vi "Agilent VNA Read Trace Display.vi"(4 "Trace":i8=1 min=1 max=99 step=1, 6 "Channel":i8=1 min=1 max=99 step=1, 7 "Agilent VNA":T1, 8 "error in (no error)":errorcluster, 11 "VISA Resource Name":refnum<visa-resource-name>) -> (0 "error out":errorcluster, 1 "Measurements":string[](array[string]), 2 "Displayed?":bool, 3 "dup VISA Resource Name":refnum<visa-resource-name>)   [LabVIEW 2011]
uses:
  TypeDefs/Agilent VNA Instrument Info.ctl
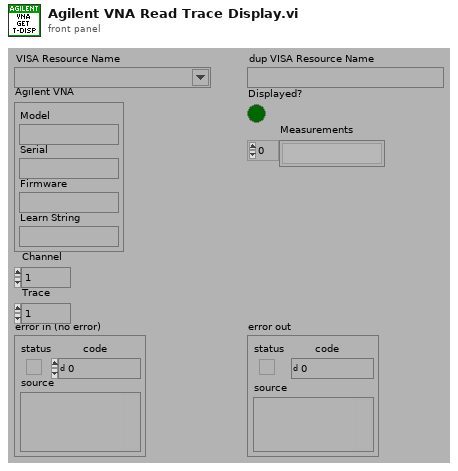
[diagram p1: front panel]
types:
  T1 = typedef "Agilent VNA Instrument Info.ctl" = cluster{"Model":string, "Serial":string, "Firmware":string, "Learn String":string}
  T2 = typedef "Agilent VNA Model.ctl" = enum16{"Not Supported", "8510X", "8719X", "8720X", "8722X", "8753X", "ENA", "PNA", "Field Fox"}
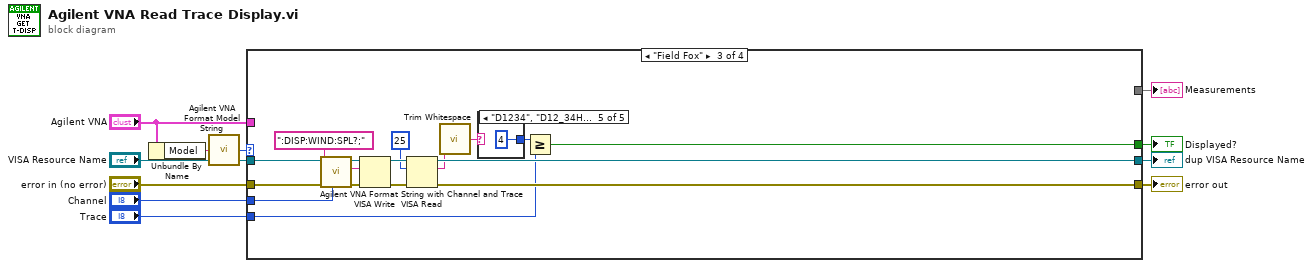
[diagram p0: block diagram]
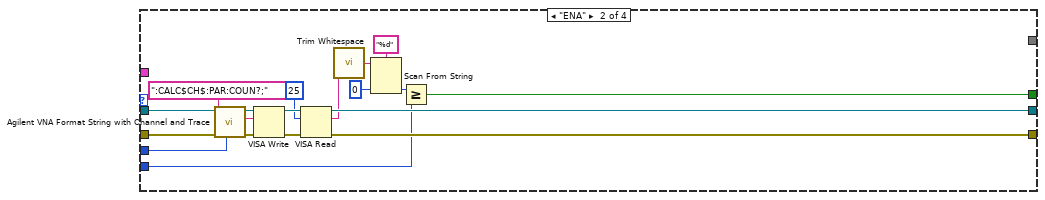
[diagram p3: hidden frame]
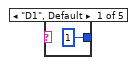
[diagram p4: hidden frame]
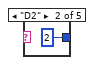
[diagram p5: hidden frame]
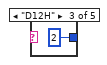
[diagram p6: hidden frame]
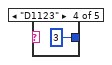
[diagram p7: hidden frame]
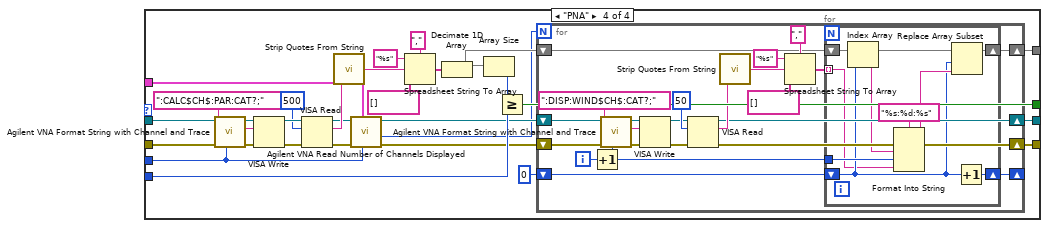
[diagram p8: hidden frame]
diagram:
  n1 = Unbundle By Name("Agilent VNA") -> ("Model"=w2:string)
  n2 = call "Agilent VNA Format Model String.vi"("Model"=w2) -> ("Model"=w7:T2)
  n3 = case shown="\"Field Fox\"" w7 {
    tunnel: "VISA Resource Name" -> [w13 w30 w45 w78]
    tunnel: "error in (no error)" -> [w12 w29 w44 w77]
    tunnel: [w13 w26 w41 w61] -> w9
    tunnel: [w12 w25 w40 w62] -> w8
    tunnel: [_ w15 w33 w64] -> w6
    tunnel: "Channel" -> [_ w20 w35 w54]
    tunnel: "Trace" -> [_ w16 w34 w68]
    tunnel: [_ _ _ w52] -> w3
    tunnel: "Agilent VNA" -> [_ _ _ w55]
    frame "Not Supported".."8753X" {
    }
    frame "ENA" {
      n4 = call "Agilent VNA Format String with Channel and Trace.vi"("Channel"=w20, "String"=":CALC$CH$:PAR:COUN?;" ("write buffer")) -> ("String Out"=w21:string)  [unwired: 1 in, 6 out]
      n5 = VISA Write(VISA resource name=w30, write buffer=w21, error in (no error)=w29) -> (VISA resource name out=w27:refnum<visa-resource-name>, error out=w28:errorcluster)  [unwired: 1 out]
      n6 = VISA Read(VISA resource name=w27, byte count=u32 25, error in (no error)=w28) -> (VISA resource name out=w26:refnum<visa-resource-name>, read buffer=w23:string, error out=w25:errorcluster)  [unwired: 1 out]
      n7 = call <vilib>:"Trim Whitespace.vi"("string"=w23) -> ("trimmed string"=w19:string)  [unwired: 1 in]
      n8 = Scan From String(format string="%d", input string=w19, default 1=i8 0 ("default value 1")) -> (output 1=w17:i8)  [unwired: 2 in, 3 out]
      n9 = Greater Or Equal?(x=w17, y=w16) -> (x >= y?=w15:bool)
    }
    frame "Field Fox" {
      n10 = call "Agilent VNA Format String with Channel and Trace.vi"("Channel"=w35, "String"=":DISP:WIND:SPL?;" ("write buffer")) -> ("String Out"=w36:string)  [unwired: 1 in, 6 out]
      n11 = VISA Write(VISA resource name=w45, write buffer=w36, error in (no error)=w44) -> (VISA resource name out=w42:refnum<visa-resource-name>, error out=w43:errorcluster)  [unwired: 1 out]
      n12 = VISA Read(VISA resource name=w42, byte count=u32 25, error in (no error)=w43) -> (VISA resource name out=w41:refnum<visa-resource-name>, read buffer=w38:string, error out=w40:errorcluster)  [unwired: 1 out]
      n13 = call <vilib>:"Trim Whitespace.vi"("string"=w38) -> ("trimmed string"=w32:string)  [unwired: 1 in]
      n14 = case shown="\"D1234\", \"D12_34H\"" w32 {
        tunnel: [i8 1 ("y") i8 2 ("y") i8 2 ("y") i8 3 ("y") i8 4 ("y")] -> w31
        frame "D1", Default {
        }
        frame "D2" {
        }
        frame "D12H" {
        }
        frame "D1123" {
        }
        frame "D1234", "D12_34H" {
        }
      }
      n15 = Greater Or Equal?(x=w31, y=w34) -> (x >= y?=w33:bool)
    }
    frame "PNA" {
      n16 = call "Agilent VNA Format String with Channel and Trace.vi"("Channel"=w54, "String"=":CALC$CH$:PAR:CAT?;" ("write buffer")) -> ("String Out"=w72:string)  [unwired: 1 in, 6 out]
      n17 = VISA Write(VISA resource name=w78, write buffer=w72, error in (no error)=w77) -> (VISA resource name out=w75:refnum<visa-resource-name>, error out=w76:errorcluster)  [unwired: 1 out]
      n18 = VISA Read(VISA resource name=w75, byte count=u32 500, error in (no error)=w76) -> (VISA resource name out=w59:refnum<visa-resource-name>, read buffer=w65:string, error out=w58:errorcluster)  [unwired: 1 out]
      n19 = call "Strip Quotes From String.vi"("String In"=w65) -> ("Trimmed String"=w66:string)
      n20 = call "Agilent VNA Read Number of Channels Displayed.vi"("Channel to be Displayed"=w54, "Agilent VNA"=w55, "error in (no error)"=w58, "VISA Resource Name"=w59) -> ("error out"=w57:errorcluster, "Channels Displayed"=w53:i8, "dup VISA Resource Name"=w56:refnum<visa-resource-name>)  [unwired: 5 out]
      n21 = Spreadsheet String To Array(delimiter (Tab)=",", format string="%s", spreadsheet string=w66, array type (2D Dbl)=string[] []) -> (array=w63:string[])
      n22 = Decimate 1D Array(w63) -> (w60:string[])  [unwired: 1 out]
      n23 = Array Size(array=w60) -> (size(s)=w67:i32)
      n24 = Greater Or Equal?(x=w67, y=w68) -> (x >= y?=w64:bool)
      n25 = for {
        N: w53 -> [_]
        shift-right: [w91] -> w62
        shift-left: w57 -> [w94]
        shift-right: [w92] -> w61
        shift-left: w56 -> [w95]
        shift-right: [w79] -> w52
        shift-left: w60 -> [w83]
        shift-right: [w80] -> _
        shift-left: 0 -> [w82]
        i -> [w89]
        n26 = Increment(x=w89) -> (x+1=w81:i32)
        n27 = call "Agilent VNA Format String with Channel and Trace.vi"("Channel"=w81, "String"=":DISP:WIND$CH$:CAT?;" ("write buffer")) -> ("String Out"=w98:string)  [unwired: 1 in, 6 out]
        n28 = VISA Write(VISA resource name=w95, write buffer=w98, error in (no error)=w94) -> (VISA resource name out=w93:refnum<visa-resource-name>, error out=w90:errorcluster)  [unwired: 1 out]
        n29 = VISA Read(VISA resource name=w93, byte count=u32 50, error in (no error)=w90) -> (VISA resource name out=w92:refnum<visa-resource-name>, read buffer=w99:string, error out=w91:errorcluster)  [unwired: 1 out]
        n30 = call "Strip Quotes From String.vi"("String In"=w99) -> ("Trimmed String"=w85:string)
        n31 = Spreadsheet String To Array(delimiter (Tab)=",", format string="%s", spreadsheet string=w85, array type (2D Dbl)=string[] []) -> (array=w84:string[])
        n32 = for {
          tunnel: w84 -> [w100] mode=indexing
          shift-right: [w107] -> w79
          shift-left: w83 -> [w108]
          tunnel: w81 -> [w104]
          shift-right: [w101] -> w80
          shift-left: w82 -> [w102]
          n33 = Index Array(array=w108, index=w102) -> (element=w105:string)
          n34 = Format Into String(format string="%s:%d:%s", w105, w104, w100) -> (resulting string=w103:string)  [unwired: 2 in, 1 out]
          n35 = Replace Array Subset(array=w108, new element=w103, index=w102) -> (w107:string[])
          n36 = Increment(x=w102) -> (x+1=w101:i32)
        }
      }
    }
  }
  "dup VISA Resource Name" <- w9
  "error out" <- w8
  "Displayed?" <- w6
  "Measurements" <- w3
